vi "Soft_Start.vi"(8 "error in (no error)":errorcluster, 10 "IMU_sample_rate":i32=200) -> (0 "error out":errorcluster, 2 "Soft Start Limits":dbl, 3 "Soft Start":bool)   [LabVIEW 2014]
uses:
  Start.vi
panel:
  out "Filter Counter":dbl
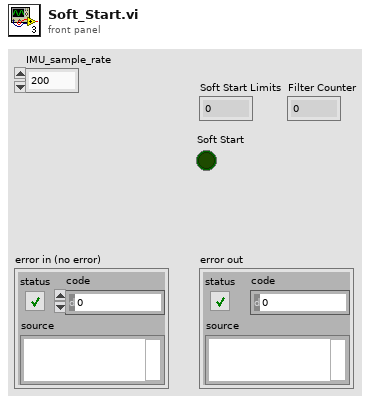
[diagram p1: front panel]
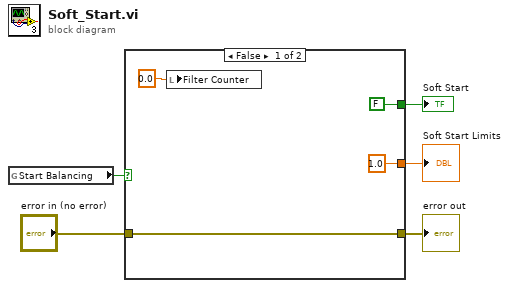
[diagram p0: block diagram]
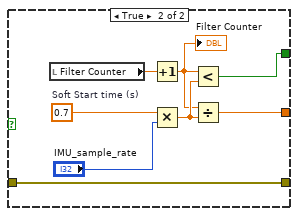
[diagram p2: hidden frame]
diagram:
  n1 = global read "Start.vi" "Start Balancing"() -> (w2:bool)
  n2 = case shown="False" w2 {
    tunnel: "error in (no error)" -> [w9 w13]
    tunnel: [w9 w13] -> w4
    tunnel: [FALSE w12] -> w1
    tunnel: [1.0 w11] -> w5
    frame False {
      n3 = local write "Filter Counter"(0.0 ("Filter Counter")) -> ()
    }
    frame True {
      w17 = 0.7  # Soft Start time (s)
      n4 = local read "Filter Counter"() -> (w10:dbl)
      n5 = Increment(x=w10) -> (x+1=w14:dbl)
      "Filter Counter" <- w14
      n6 = Multiply(x=w17, y="IMU_sample_rate") -> (x*y=w15:dbl)
      n7 = Less?(x=w14, y=w15) -> (x < y?=w12:bool)
      n8 = Divide(x=w14, y=w15) -> (x/y=w11:dbl)
    }
  }
  "Soft Start Limits" <- w5
  "error out" <- w4
  "Soft Start" <- w1
